vi "Write Needed Points.vi"(8 "error in (no error)":errorcluster, 10 "Needed Points":T1(array[ring]), 11 "PathCommands in":refnum<class "PathCommands.lvclass">) -> (0 "error out":errorcluster, 3 "PathCommands out":refnum<class "PathCommands.lvclass">)   [LabVIEW 2019, in "PathCommands.lvclass"]
uses:
  PathCommands.lvclass
  PathCommands.lvclass/PathCommands.ctl
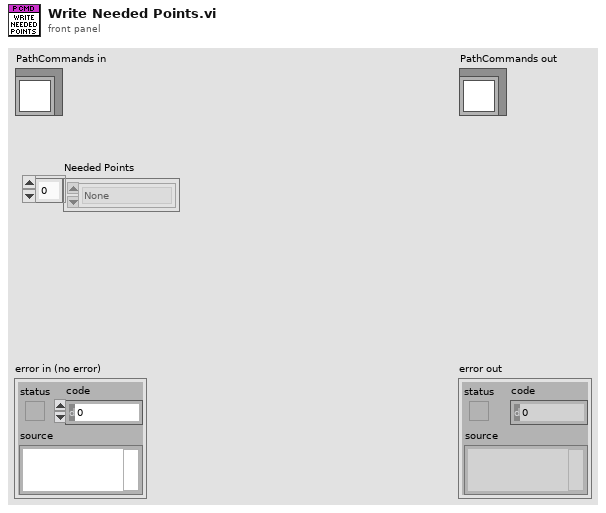
[diagram p1: front panel]
types:
  T1 = enum16{"None", "After", "Before", "Last", "First"}[]
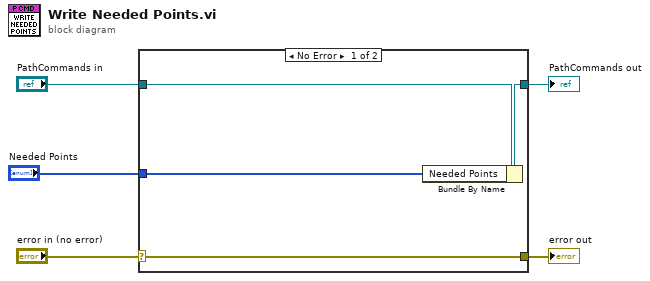
[diagram p0: block diagram]
diagram:
  n1 = case shown="No Error" "error in (no error)" {
    selector: "error in (no error)" -> [w9 w10]
    tunnel: [w9 w10] -> w4
    tunnel: [w7 w11] -> w2
    tunnel: "PathCommands in" -> [w8 w11]
    tunnel: "Needed Points" -> [w6 _]
    frame No Error {
      n2 = Bundle By Name(cluster=w8, "Needed Points"=w6) -> (w7:refnum<class "PathCommands.lvclass">)
    }
    frame Error {
    }
  }
  "error out" <- w4
  "PathCommands out" <- w2
